vi "serialClose.vi"(8 "error in (no error)":errorcluster, 11 "Python in":T1) -> (0 "error out":errorcluster)   [LabVIEW 2019]
uses:
  Past SmartMotor UI Iterations/SerialVIs/PythonCtrl.ctl
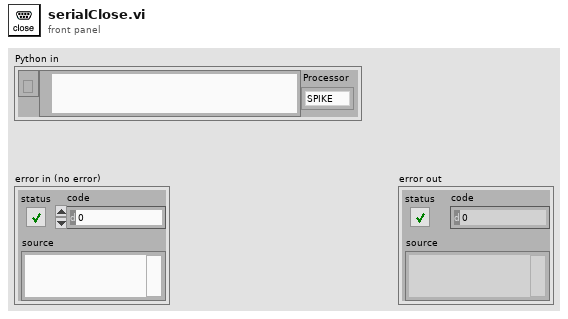
[diagram p1: front panel]
types:
  T1 = typedef "PythonCtrl.ctl" = cluster{"session":refnum<k35>, "PyPath":path, "Processor":enum16{"SPIKE", "Pi", "Pi_ssh"}}
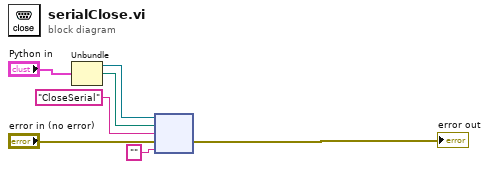
[diagram p0: block diagram]
diagram:
  n1 = Unbundle("Python in") -> ("session"=w2:refnum<k35>, "PyPath"=w1:path)  [unwired: 1 out]
  n2 = node(w2, w1, "CloseSerial" ("function name"), "error in (no error)", "" ("function name")) -> (→"error out":errorcluster)  [unwired: 1 in, 3 out]
